vi "Parse Result.vi"(8 "error in (no error)":errorcluster, 9 "Number of Parameters":u32, 10 "Raw Result":string, 11 "Driver in":refnum<class "Driver.lvclass">) -> (0 "error out":errorcluster, 1 "Parameter Raw Result":string[](array[string]), 2 "Command Raw Result":string, 3 "Driver out":refnum<class "Driver.lvclass">)   [LabVIEW 2023, in "HAF.lvlib" / "Driver.lvclass"]
doc: "Parses a result from an Instrument into its Command and Parameter(s) constituents.  Subclasses should override this where instrument specific variation occurs. \n\nThe parent implementation assumes the following:\n* If no parameters are used then the result is solely for the Command\n* The result is tokenised on “,”\n* If parameters are used, and the number of tokens = num parameters, result is solely for the parameters\n* If the number of tokens = num parameters + 1, the first token is for the Command and the reminaing for parameters.\n* Parameter tokens are loaded, in order, to a parameter array.\n\nThe Command is responsible for dealing with the Command Raw Result and Parameter Raw Result array."
uses:
  Driver.lvclass
  Driver.lvclass/Driver.ctl
  HAF.lvlib
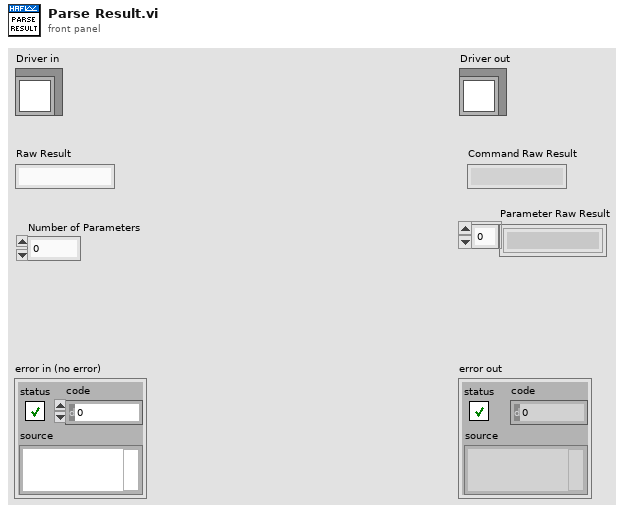
[diagram p1: front panel]
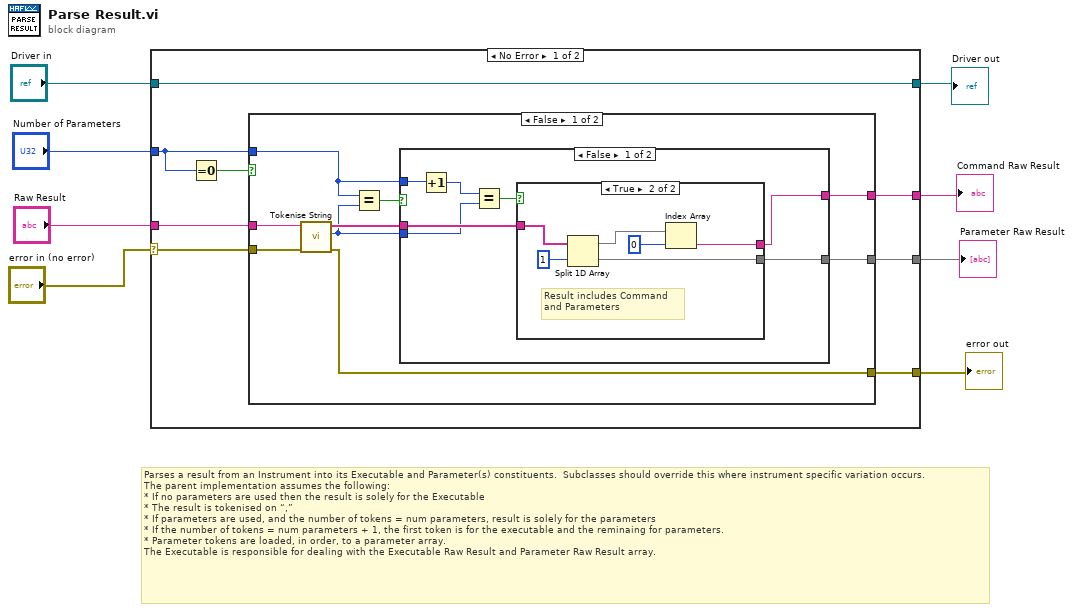
[diagram p0: block diagram]
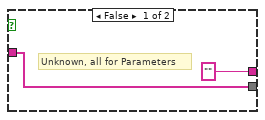
[diagram p2: hidden frame]
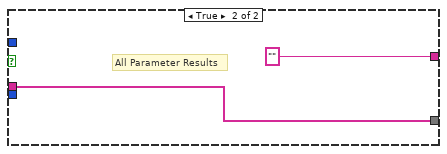
[diagram p3: hidden frame]
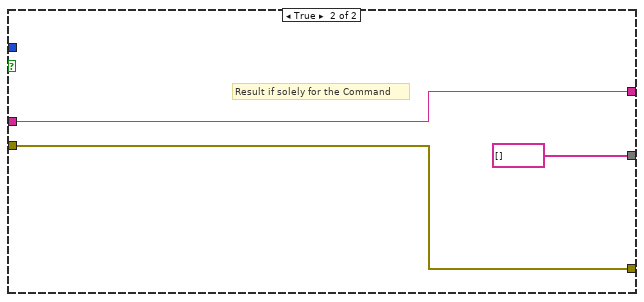
[diagram p4: hidden frame]
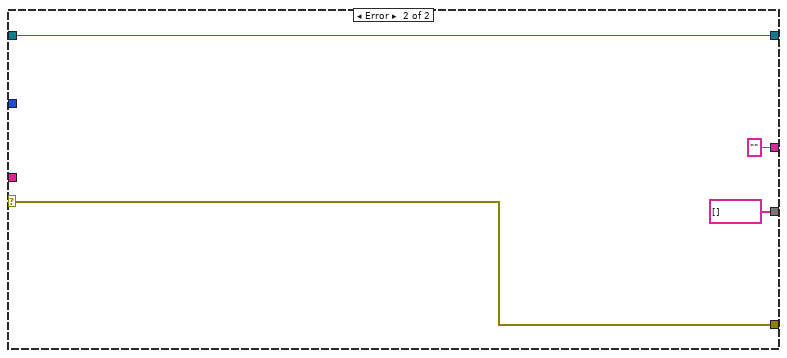
[diagram p5: hidden frame]
diagram:
  # "Parses a result from an Instrument into its Executable and Parameter(s) constituents.  Subclasses should override this where instrument specific variation occurs. \nThe parent implementation assumes the following:\n* If no parameters are used then the result is solely for the Executable\n* The result is tokenised on “,”\n* If parameters are used, and the number of tokens = num parameters, result is solely for the parameters\n* If the number of tokens = num parameters + 1, the first token is for the executable and the reminaing for parameters.\n* Parameter tokens are loaded, in order, to a parameter array.\nThe Executable is responsible for dealing with the Executable Raw Result and Parameter Raw Result array."
  n1 = case shown="No Error" "error in (no error)" {
    selector: "error in (no error)" -> [w12 w49]
    tunnel: [w11 w49] -> w1
    tunnel: [w16 w48] -> w6
    tunnel: "Driver in" -> [w16 w48]
    tunnel: "Number of Parameters" -> [w15 _]
    tunnel: "Raw Result" -> [w13 _]
    tunnel: [w10 "" ("Raw Result")] -> w3
    tunnel: [w9 string[] [] ("Tokens")] -> w2
    frame No Error {
      n2 = Equal To 0?(x=w15) -> (x = 0?=w14:bool)
      n3 = case shown="False" w14 {
        tunnel: w15 -> [w22 _]
        tunnel: w13 -> [w25 w45]
        tunnel: w12 -> [w24 w43]
        tunnel: [w18 w45] -> w10
        tunnel: [w17 string[] []] -> w9
        tunnel: [w19 w43] -> w11
        frame False {
          n4 = call "Tokenise String.vi"("error in (no error)"=w24, "String to Parse"=w25) -> ("error out"=w19:errorcluster, "Token Count"=w20:i32, "Tokens"=w21:string[])  [unwired: 6 in, 1 out]
          n5 = Equal?(x=w22, y=w20) -> (x = y?=w23:bool)
          n6 = case shown="False" w23 {
            tunnel: [w27 ""] -> w18
            tunnel: w22 -> [w32 _]
            tunnel: w21 -> [w29 w41]
            tunnel: [w26 w41] -> w17
            tunnel: w20 -> [w28 _]
            frame False {
              n7 = Increment(x=w32) -> (x+1=w31:u32)
              n8 = Equal?(x=w31, y=w28) -> (x = y?=w30:bool)
              n9 = case shown="True" w30 {
                tunnel: w29 -> [w34 w40]
                tunnel: ["" ("String") w36] -> w27
                tunnel: [w34 w35] -> w26
                frame False {
                  # "Unknown, all for Parameters"
                }
                frame True {
                  # "Result includes Command\nand Parameters"
                  n10 = Split 1D Array(array=w40, index=1) -> (first subarray=w38:string[], second subarray=w35:string[])
                  n11 = Index Array(array=w38, index=0) -> (element=w36:string)
                }
              }
            }
            frame True {
              # "All Parameter Results"
            }
          }
        }
        frame True {
          # "Result if solely for the Command"
        }
      }
    }
    frame Error {
    }
  }
  "error out" <- w1
  "Driver out" <- w6
  "Command Raw Result" <- w3
  "Parameter Raw Result" <- w2
